vi "Read Packet Identifier.vi"(11 "ControlPacket in":refnum<class "ControlPacket.lvclass">) -> (2 "Packet Identifier":u16 format="%016b", 3 "ControlPacket out":refnum<class "ControlPacket.lvclass">)   [LabVIEW 2013, in "ControlPacket.lvclass"]
uses:
  ControlPacket.lvclass
  ControlPacket.lvclass/ControlPacket.ctl
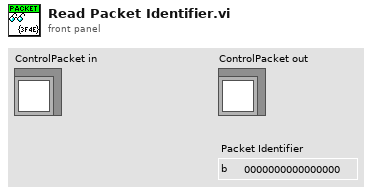
[diagram p1: front panel]
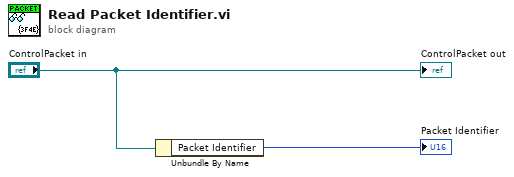
[diagram p0: block diagram]
diagram:
  n1 = Unbundle By Name("ControlPacket in") -> ("Packet Identifier"=→"Packet Identifier":u16)
  "ControlPacket out" <- "ControlPacket in"
